vi "GLOBAL Experiment Metadata.vi"() -> ()   [LabVIEW 2018]
panel:
  in  "Laser power (W)":dbl
  in  "Stage":cluster{"X (mm)":dbl, "Y (mm)":dbl}
  in  "Illumination":T1
  in  "Hardware Configuration":string
  in  "Software Version":string
  # "Use this VI for storing metadata for saving into movie files.\nSee Virtual Camera/Create Stack Info.vi"
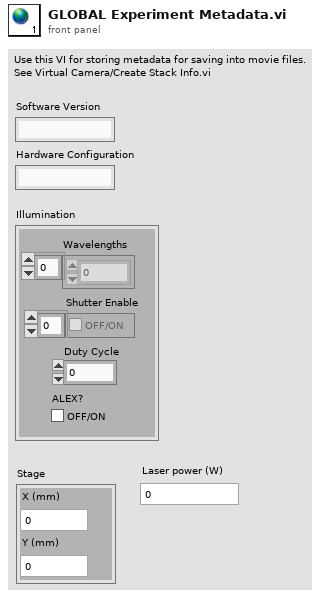
[diagram p1: front panel]
types:
  T1 = cluster{"Shutter Enable":bool[], "Duty Cycle":dbl, "Wavelengths":dbl[], "ALEX?":bool}
diagram:
